vi "Autonomous Independent.vi"   [LabVIEW 2020]
doc: "This VI is called when autonomous begins, and will automatically be terminated when autonomous ends. You can carry out timed or sensor driven robot movement independently without needing to return to the caller."
uses:
  <vilib>/Rock Robotics/WPI/Utilities/WPI_GetSetVariantRefNum.vi
  <vilib>/Rock Robotics/Network Tables/NT Read String.vi
  <vilib>/Rock Robotics/Network Tables/NT Write Numeric Array.vi
  <vilib>/Rock Robotics/WPI/RobotDrive/WPI_RobotDriveArcadeDrive_Standard(NoSaturation).vi
panel:
  # "Be sure to right-click and choose Data Operations>>Make Current Value default if you want to save the array values with the VI"
types:
  T1 = typedef "WPI_JoystickDevRef.ctl" = cluster{"Device":T2}
  T2 = typedef "WPI_JoystickDeviceEnum.ctl" = enum16{"USB 0", "USB 1", "USB 2", "USB 3", "USB 4", "USB 5"}
  T3 = typedef "WPI_RobotDriveDevRef.ctl" = cluster{"DevStatus":errorcluster, "Motors[]":T4[], "Square Inputs":bool, "Max Output":dbl}
  T4 = typedef "WPI_MotorControlDeviceRef.ctl" = cluster{"DeviceStatus":errorcluster, "Type":T5, "PWM":cluster{"PWM Channel":T6, "DeadBand":T7}, "CAN":cluster{"Device Number":u8, "SetOutput VI Ref":variant, "GetOutput VI Ref":variant, "Enable VI Ref":variant, "Disable VI Ref":variant, "Data":variant}, "Invert":bool, "DIO PWM":cluster{"PWM \"Enable\" Channel":T6, "DIOChannel":T8, "PWM Rate":dbl}}
  T5 = typedef "WPI_MotorControlType.ctl" = enum16{"PWM", "CAN", "DIO PWM"}
  T6 = typedef "FPGA_DIOPWMChannel.ctl" = enum8{"PWM 0", "PWM 1", "PWM 2", "PWM 3", "PWM 4", "PWM 5", "PWM 6", "PWM 7", "PWM 8", "PWM 9", "PWM MXP 0", "PWM MXP 1", "PWM MXP 2", "PWM MXP 3", "PWM MXP 4", "PWM MXP 5", "PWM MXP 6", "PWM MXP 7", "PWM MXP 8", "PWM MXP 9", "Invalid"}
  T7 = typedef "WPI_PWMDeadband.ctl" = cluster{"Name":string, "maxPositivePwm":i32, "minPositivePwm":i32, "centerPwm":i32, "maxNegativePwm":i32, "minNegativePwm":i32, "angularRange":u16}
  T8 = typedef "FPGA_DIOChannel.ctl" = enum8{"DIO 0", "DIO 1", "DIO 2", "DIO 3", "DIO 4", "DIO 5", "DIO 6", "DIO 7", "DIO 8", "DIO 9", "DIO MXP 0", "DIO MXP 1", "DIO MXP 2", "DIO MXP 3", "DIO MXP 4", "DIO MXP 5", "DIO MXP 6", "DIO MXP 7", "DIO MXP 8", "DIO MXP 9", "DIO MXP 10", "DIO MXP 11", "DIO MXP 12", "DIO MXP 13", "DIO MXP 14", "DIO MXP 15", "SPI Port CS1", "SPI Port CS2", "SPI Port CS3", "SPI Port MISO", "SPI Port MOSI", "Invalid"}
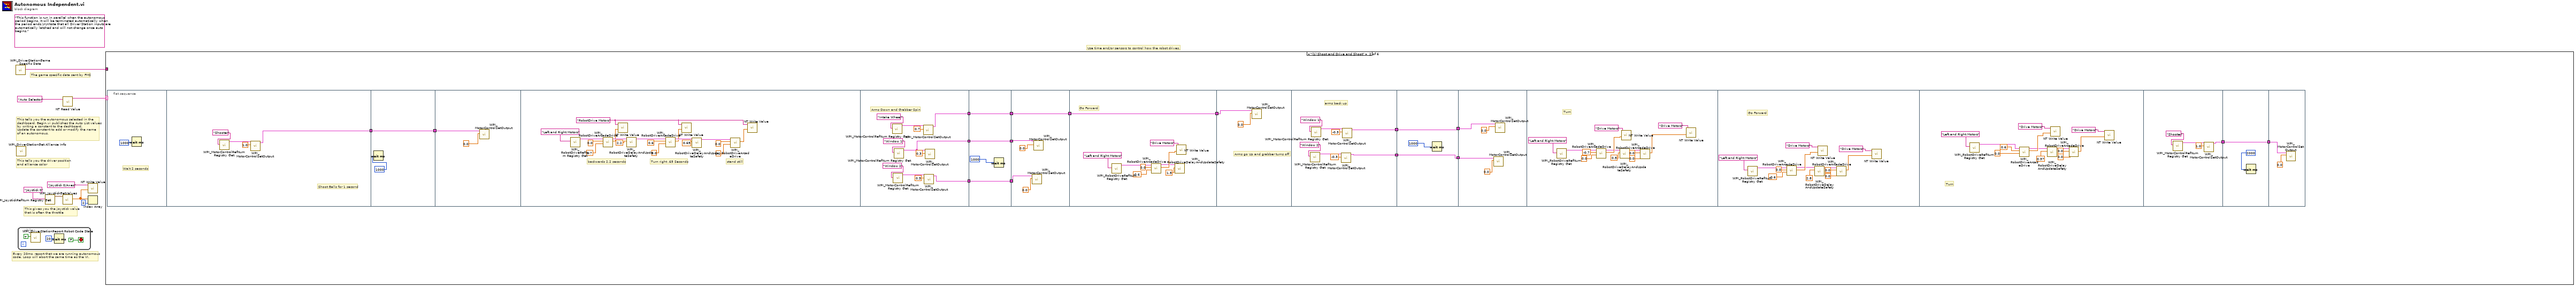
[diagram p0: block diagram]
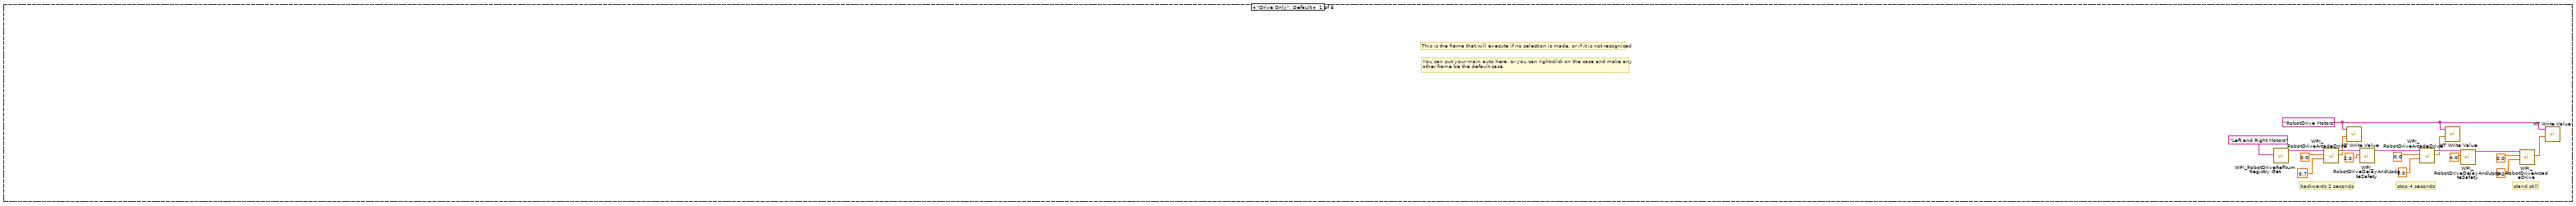
[diagram p2: hidden frame]
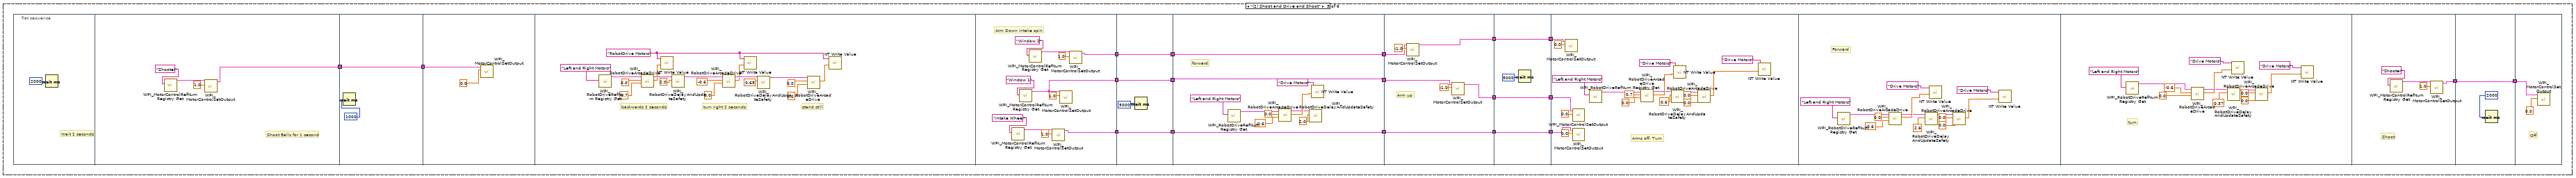
[diagram p3: hidden frame]
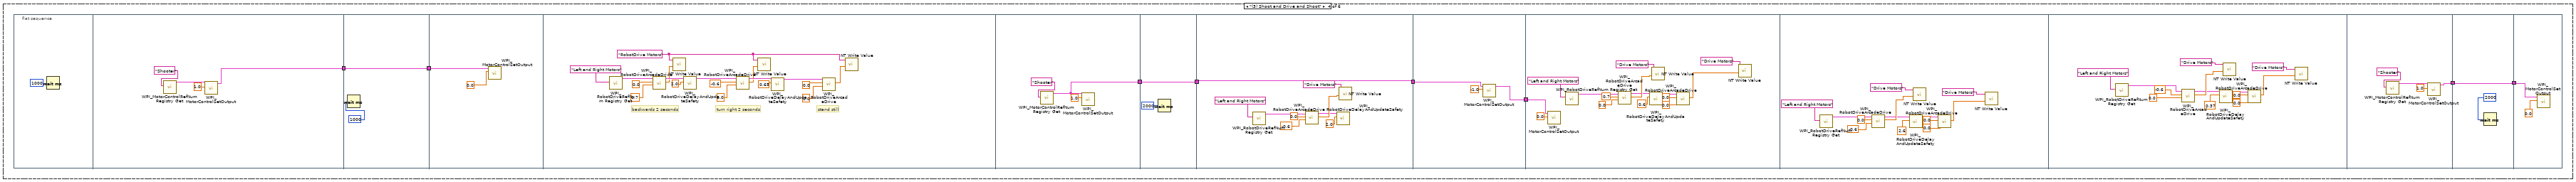
[diagram p4: hidden frame]
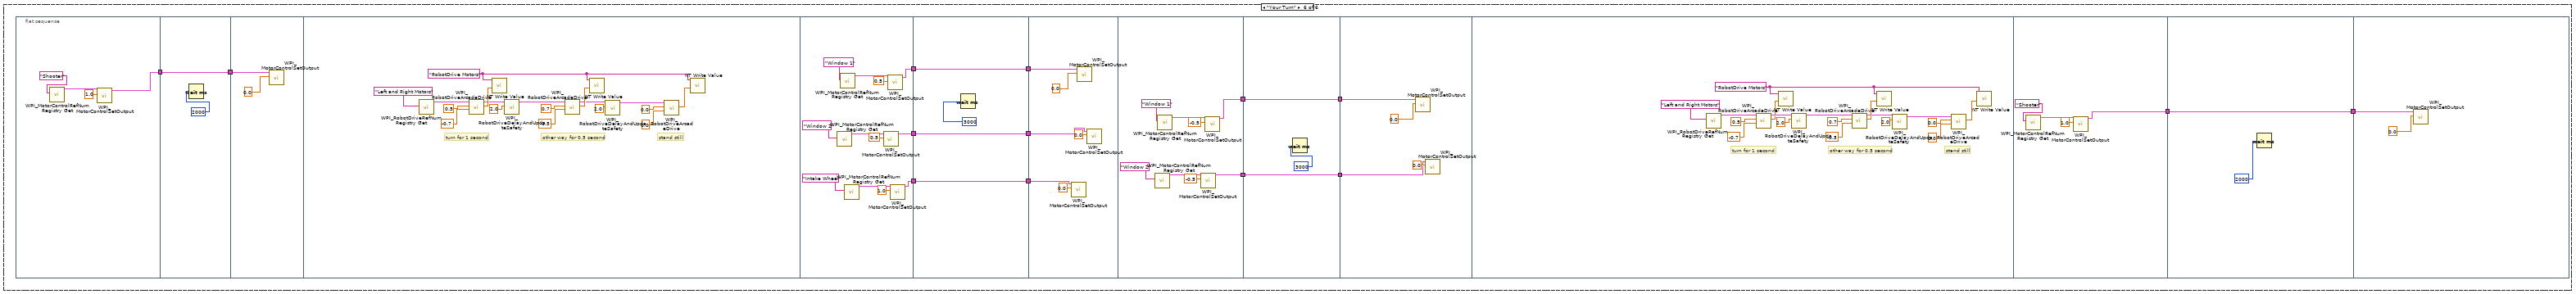
[diagram p6: hidden frame]
diagram:
  (unwired) "This function is run in parallel when the autonomous period begins. It will be terminated automatically when the period ends.\n\nNote that all Driver Station inputs are automatically latched and will not change once auto begins."
  # "The game specific data sent by FMS"
  # "This tells you the autonomous selected in the \ndashboard. Begin.vi publishes the Auto List values\nby writing a constant to the dashboard.\nUpdate the constant to add or modify the name\nof an autonomous."
  # "Every 20ms, report that we are running autonomous\ncode. Loop will abort the same time as the VI."
  # "This gives you the joystick value\nthat is often the throttle"
  # "Use time and/or sensors to control how the robot drives."
  # "This tells you the driver position\nand alliance color"
  n1 = call <vilib>:"WPI_DriverStationGame Specific Data.vi"() -> ("Game Specific Data"=w1:string)  [unwired: 11 in]
  n2 = call <vilib>:"WPI_DriverStationGet Alliance Info.vi"() -> ()  [unwired: 12 out]
  n3 = while {
    stop <- FALSE stop-if-true
    n4 = call <vilib>:"WPI_DriverStationReport Robot Code State.vi"("Autonomous"=TRUE) -> ()  [unwired: 10 in, 1 out]
    n5 = Wait (ms)(milliseconds to wait=u32 20) -> ()  [unwired: 1 out]
  }
  n6 = call <vilib>:"WPI_JoystickRefNum Registry Get.vi"("refnum name"="Joystick 0") -> ("JoystickDevRef"=w7:T1)  [unwired: 1 in, 9 out]
  n7 = call <vilib>:"WPI_JoystickGetValues.vi"("JoystickDevRef"=w7) -> ("Axes"=w3:dbl[])  [unwired: 6 in, 4 out]
  n8 = call-poly <vilib>:"NT Read Value.vi"("Name"="Auto Selector") -> ("String"=w4:string)  [unwired: 9 in, 1 out]
  n9 = call-poly <vilib>:"NT Write Value.vi"("Numeric Array"=w3, "Name"="Joystick 0/Axes") -> ()  [unwired: 9 in, 1 out]
  n10 = Index Array(array=w3, index=2) -> ()  [unwired: 1 out]
  n11 = case shown="\"(1) Shoot and Drive and Shoot\"" w4 {
    tunnel: w1 -> [_ _ _ _ _ _]
    frame "Drive Only", Default {
      w14 = "RobotDrive Motors" ("Name")
      # "stand still"
      # "stop 4 seconds"
      # "backwards 2 seconds"
      # "You can put your main auto here, or you can right-click on the case and make any\nother frame be the default case."
      # "This is the frame that will execute if no selection is made, or if it is not recognized"
      n12 = call <vilib>:"WPI_RobotDriveRefNum Registry Get.vi"("refnum name"="Left and Right Motors") -> ("RobotDriveDevRef"=w29:T3)  [unwired: 1 in, 9 out]
      n13 = call-poly <vilib>:"WPI_RobotDriveArcadeDrive.vi"("Y axis value"=0.7 ("X axis value"), "X axis value"=0.0, "RobotDriveDevRef"=w29) -> ("Motor Values"=w13:dbl[], "RobotDriveDevRef"=w23:T3)  [unwired: 1 in, 6 out]
      n14 = call-poly <vilib>:"NT Write Value.vi"("Numeric Array"=w13, "Name"=w14) -> ()  [unwired: 9 in, 1 out]
      n15 = call <vilib>:"WPI_RobotDriveDelayAndUpdateSafety.vi"("Delay (s)"=2.0, "RobotDriveDevRef"=w23) -> ("RobotDriveDevRef 2"=w12:T3)  [unwired: 8 in, 1 out]
      n16 = call-poly <vilib>:"WPI_RobotDriveArcadeDrive.vi"("Y axis value"=0.0 ("X axis value"), "X axis value"=0.0, "RobotDriveDevRef"=w12) -> ("Motor Values"=w15:dbl[], "RobotDriveDevRef"=w24:T3)  [unwired: 1 in, 6 out]
      n17 = call-poly <vilib>:"NT Write Value.vi"("Numeric Array"=w15, "Name"=w14) -> ()  [unwired: 9 in, 1 out]
      n18 = call <vilib>:"WPI_RobotDriveDelayAndUpdateSafety.vi"("Delay (s)"=4.0, "RobotDriveDevRef"=w24) -> ("RobotDriveDevRef 2"=w25:T3)  [unwired: 8 in, 1 out]
      n19 = call-poly <vilib>:"WPI_RobotDriveArcadeDrive.vi"("Y axis value"=0.0 ("X axis value"), "X axis value"=0.0, "RobotDriveDevRef"=w25) -> ("Motor Values"=w16:dbl[])  [unwired: 1 in, 7 out]
      n20 = call-poly <vilib>:"NT Write Value.vi"("Numeric Array"=w16, "Name"=w14) -> ()  [unwired: 9 in, 1 out]
    }
    frame "(1) Shoot and Drive and Shoot" {
      n21 = flat-sequence {
        tunnel: [w47] -> w45
        tunnel: w45 -> [w51]
        tunnel: [w51] -> w44
        tunnel: w44 -> [w53]
        tunnel: [w81] -> w43
        tunnel: [w77] -> w40
        tunnel: [w73] -> w38
        tunnel: w43 -> [w85]
        tunnel: w40 -> [w84]
        tunnel: [w86] -> w37
        tunnel: w38 -> [w86]
        tunnel: [w85] -> w35
        tunnel: [w84] -> w34
        tunnel: w37 -> [w92]
        tunnel: [w92] -> w36
        tunnel: w35 -> [w91]
        tunnel: w34 -> [w89]
        tunnel: [w93] -> w39
        tunnel: w36 -> [w93]
        tunnel: w39 -> [w103]
        tunnel: [w105] -> w32
        tunnel: [w104] -> w31
        tunnel: [w113] -> w33
        tunnel: w32 -> [w113]
        tunnel: w31 -> [w112]
        tunnel: [w112] -> w30
        tunnel: w33 -> [w116]
        tunnel: w30 -> [w115]
        tunnel: [w158] -> w41
        tunnel: [w162] -> w42
        tunnel: w41 -> [w162]
        tunnel: w42 -> [w164]
        frame #0 {
          # "Wait 2 seconds"
          n22 = Wait (ms)(milliseconds to wait=u32 1000) -> ()  [unwired: 1 out]
        }
        frame #1 {
          # "Shoot Balls for 1 second"
          n23 = call <vilib>:"WPI_MotorControlRefNum Registry Get.vi"("refnum name"="Shooter") -> ("MotorControlDevRef"=w50:T4)  [unwired: 9 in, 1 out]
          n24 = call <vilib>:"WPI_MotorControlSetOutput.vi"("Output"=1.0, "MotorControlDevRef"=w50) -> ("MotorControlDevRef"=w47:T4)  [unwired: 7 in, 2 out]
        }
        frame #2 {
          n25 = Wait (ms)(milliseconds to wait=u32 1000) -> ()  [unwired: 1 out]
        }
        frame #3 {
          n26 = call <vilib>:"WPI_MotorControlSetOutput.vi"("Output"=0.0, "MotorControlDevRef"=w53) -> ()  [unwired: 7 in, 3 out]
        }
        frame #4 {
          w57 = "RobotDrive Motors" ("Name")
          # "stand still"
          # "Turn right .65 Seconds"
          # "backwards 2.2 seconds"
          n27 = call <vilib>:"WPI_RobotDriveRefNum Registry Get.vi"("refnum name"="Left and Right Motors") -> ("RobotDriveDevRef"=w72:T3)  [unwired: 1 in, 9 out]
          n28 = call-poly <vilib>:"WPI_RobotDriveArcadeDrive.vi"("Y axis value"=0.7 ("X axis value"), "X axis value"=0.0, "RobotDriveDevRef"=w72) -> ("Motor Values"=w56:dbl[], "RobotDriveDevRef"=w66:T3)  [unwired: 1 in, 6 out]
          n29 = call-poly <vilib>:"NT Write Value.vi"("Numeric Array"=w56, "Name"=w57) -> ()  [unwired: 9 in, 1 out]
          n30 = call <vilib>:"WPI_RobotDriveDelayAndUpdateSafety.vi"("Delay (s)"=2.2, "RobotDriveDevRef"=w66) -> ("RobotDriveDevRef 2"=w55:T3)  [unwired: 8 in, 1 out]
          n31 = call-poly <vilib>:"WPI_RobotDriveArcadeDrive.vi"("Y axis value"=0.0 ("X axis value"), "X axis value"=0.6, "RobotDriveDevRef"=w55) -> ("Motor Values"=w58:dbl[], "RobotDriveDevRef"=w67:T3)  [unwired: 1 in, 6 out]
          n32 = call-poly <vilib>:"NT Write Value.vi"("Numeric Array"=w58, "Name"=w57) -> ()  [unwired: 9 in, 1 out]
          n33 = call <vilib>:"WPI_RobotDriveDelayAndUpdateSafety.vi"("Delay (s)"=0.65, "RobotDriveDevRef"=w67) -> ("RobotDriveDevRef 2"=w68:T3)  [unwired: 8 in, 1 out]
          n34 = call-poly <vilib>:"WPI_RobotDriveArcadeDrive.vi"("Y axis value"=0.0 ("X axis value"), "X axis value"=0.0, "RobotDriveDevRef"=w68) -> ("Motor Values"=w59:dbl[])  [unwired: 1 in, 7 out]
          n35 = call-poly <vilib>:"NT Write Value.vi"("Numeric Array"=w59, "Name"=w57) -> ()  [unwired: 9 in, 1 out]
        }
        frame #5 {
          # "Arms Down and Grabber Spin"
          n36 = call <vilib>:"WPI_MotorControlRefNum Registry Get.vi"("refnum name"="Intake Wheel") -> ("MotorControlDevRef"=w74:T4)  [unwired: 9 in, 1 out]
          n37 = call <vilib>:"WPI_MotorControlRefNum Registry Get.vi"("refnum name"="Window 2") -> ("MotorControlDevRef"=w79:T4)  [unwired: 9 in, 1 out]
          n38 = call <vilib>:"WPI_MotorControlRefNum Registry Get.vi"("refnum name"="Window 1") -> ("MotorControlDevRef"=w81:T4)  [unwired: 9 in, 1 out]
          n39 = call <vilib>:"WPI_MotorControlSetOutput.vi"("Output"=0.7, "MotorControlDevRef"=w74) -> ("MotorControlDevRef"=w73:T4)  [unwired: 7 in, 2 out]
          n40 = call <vilib>:"WPI_MotorControlSetOutput.vi"("Output"=0.3, "MotorControlDevRef"=w79) -> ("MotorControlDevRef"=w77:T4)  [unwired: 7 in, 2 out]
          n41 = call <vilib>:"WPI_MotorControlSetOutput.vi"("Output"=0.3, "MotorControlDevRef"=w81) -> ()  [unwired: 7 in, 3 out]
        }
        frame #6 {
          n42 = Wait (ms)(milliseconds to wait=u32 1000) -> ()  [unwired: 1 out]
        }
        frame #7 {
          n43 = call <vilib>:"WPI_MotorControlSetOutput.vi"("Output"=0.0, "MotorControlDevRef"=w89) -> ()  [unwired: 7 in, 3 out]
          n44 = call <vilib>:"WPI_MotorControlSetOutput.vi"("Output"=0.0, "MotorControlDevRef"=w91) -> ()  [unwired: 7 in, 3 out]
        }
        frame #8 {
          # "Go Forward"
          n45 = call <vilib>:"WPI_RobotDriveRefNum Registry Get.vi"("refnum name"="Left and Right Motors") -> ("RobotDriveDevRef"=w101:T3)  [unwired: 9 in, 1 out]
          n46 = call-poly <vilib>:"WPI_RobotDriveArcadeDrive.vi"("Y axis value"=-0.6, "X axis value"=0.0, "RobotDriveDevRef"=w101) -> ("Motor Values"=w100:dbl[], "RobotDriveDevRef"=w97:T3)  [unwired: 6 in, 1 out]
          n47 = call <vilib>:"WPI_RobotDriveDelayAndUpdateSafety.vi"("Delay (s)"=1.5, "RobotDriveDevRef"=w97) -> ()  [unwired: 8 in, 2 out]
          n48 = call-poly <vilib>:"NT Write Value.vi"("Numeric Array"=w100, "Name"="Drive Motors") -> ()  [unwired: 9 in, 1 out]
        }
        frame #9 {
          # "Arms go Up and grabber turns off"
          n49 = call <vilib>:"WPI_MotorControlSetOutput.vi"("Output"=0.0, "MotorControlDevRef"=w103) -> ()  [unwired: 7 in, 3 out]
        }
        frame #10 {
          # "arms back up"
          n50 = call <vilib>:"WPI_MotorControlRefNum Registry Get.vi"("refnum name"="Window 2") -> ("MotorControlDevRef"=w107:T4)  [unwired: 9 in, 1 out]
          n51 = call <vilib>:"WPI_MotorControlRefNum Registry Get.vi"("refnum name"="Window 1") -> ("MotorControlDevRef"=w109:T4)  [unwired: 9 in, 1 out]
          n52 = call <vilib>:"WPI_MotorControlSetOutput.vi"("Output"=-0.3, "MotorControlDevRef"=w107) -> ("MotorControlDevRef"=w104:T4)  [unwired: 7 in, 2 out]
          n53 = call <vilib>:"WPI_MotorControlSetOutput.vi"("Output"=-0.3, "MotorControlDevRef"=w109) -> ("MotorControlDevRef"=w105:T4)  [unwired: 7 in, 2 out]
        }
        frame #11 {
          n54 = Wait (ms)(milliseconds to wait=u32 1000) -> ()  [unwired: 1 out]
        }
        frame #12 {
          n55 = call <vilib>:"WPI_MotorControlSetOutput.vi"("Output"=0.0, "MotorControlDevRef"=w115) -> ()  [unwired: 7 in, 3 out]
          n56 = call <vilib>:"WPI_MotorControlSetOutput.vi"("Output"=0.0, "MotorControlDevRef"=w116) -> ()  [unwired: 7 in, 3 out]
        }
        frame #13 {
          # "Turn"
          n57 = call <vilib>:"WPI_RobotDriveRefNum Registry Get.vi"("refnum name"="Left and Right Motors") -> ("RobotDriveDevRef"=w131:T3)  [unwired: 9 in, 1 out]
          n58 = call-poly <vilib>:"WPI_RobotDriveArcadeDrive.vi"("Y axis value"=0.0, "X axis value"=-0.7, "RobotDriveDevRef"=w131) -> ("Motor Values"=w130:dbl[], "RobotDriveDevRef"=w128:T3)  [unwired: 6 in, 1 out]
          n59 = call <vilib>:"WPI_RobotDriveDelayAndUpdateSafety.vi"("Delay (s)"=0.5, "RobotDriveDevRef"=w128) -> ("RobotDriveDevRef 2"=w124:T3)  [unwired: 8 in, 1 out]
          n60 = call-poly <vilib>:"NT Write Value.vi"("Numeric Array"=w130, "Name"="Drive Motors") -> ()  [unwired: 9 in, 1 out]
          n61 = call-poly <vilib>:"WPI_RobotDriveArcadeDrive.vi"("Y axis value"=0.0, "X axis value"=0.0, "RobotDriveDevRef"=w124) -> ("Motor Values"=w121:dbl[])  [unwired: 6 in, 2 out]
          n62 = call-poly <vilib>:"NT Write Value.vi"("Numeric Array"=w121, "Name"="Drive Motors") -> ()  [unwired: 9 in, 1 out]
        }
        frame #14 {
          # "Go Forward"
          n63 = call <vilib>:"WPI_RobotDriveRefNum Registry Get.vi"("refnum name"="Left and Right Motors") -> ("RobotDriveDevRef"=w144:T3)  [unwired: 9 in, 1 out]
          n64 = call-poly <vilib>:"WPI_RobotDriveArcadeDrive.vi"("Y axis value"=-0.6, "X axis value"=0.0, "RobotDriveDevRef"=w144) -> ("Motor Values"=w143:dbl[], "RobotDriveDevRef"=w141:T3)  [unwired: 6 in, 1 out]
          n65 = call <vilib>:"WPI_RobotDriveDelayAndUpdateSafety.vi"("Delay (s)"=2.8, "RobotDriveDevRef"=w141) -> ("RobotDriveDevRef 2"=w136:T3)  [unwired: 8 in, 1 out]
          n66 = call-poly <vilib>:"NT Write Value.vi"("Numeric Array"=w143, "Name"="Drive Motors") -> ()  [unwired: 9 in, 1 out]
          n67 = call-poly <vilib>:"WPI_RobotDriveArcadeDrive.vi"("Y axis value"=0.0, "X axis value"=0.0, "RobotDriveDevRef"=w136) -> ("Motor Values"=w132:dbl[])  [unwired: 6 in, 2 out]
          n68 = call-poly <vilib>:"NT Write Value.vi"("Numeric Array"=w132, "Name"="Drive Motors") -> ()  [unwired: 9 in, 1 out]
        }
        frame #15 {
          # "Turn"
          n69 = call <vilib>:"WPI_RobotDriveRefNum Registry Get.vi"("refnum name"="Left and Right Motors") -> ("RobotDriveDevRef"=w157:T3)  [unwired: 9 in, 1 out]
          n70 = call-poly <vilib>:"WPI_RobotDriveArcadeDrive.vi"("Y axis value"=0.0, "X axis value"=0.6, "RobotDriveDevRef"=w157) -> ("Motor Values"=w156:dbl[], "RobotDriveDevRef"=w154:T3)  [unwired: 6 in, 1 out]
          n71 = call <vilib>:"WPI_RobotDriveDelayAndUpdateSafety.vi"("Delay (s)"=0.37, "RobotDriveDevRef"=w154) -> ("RobotDriveDevRef 2"=w149:T3)  [unwired: 8 in, 1 out]
          n72 = call-poly <vilib>:"NT Write Value.vi"("Numeric Array"=w156, "Name"="Drive Motors") -> ()  [unwired: 9 in, 1 out]
          n73 = call-poly <vilib>:"WPI_RobotDriveArcadeDrive.vi"("Y axis value"=0.0, "X axis value"=0.0, "RobotDriveDevRef"=w149) -> ("Motor Values"=w145:dbl[])  [unwired: 6 in, 2 out]
          n74 = call-poly <vilib>:"NT Write Value.vi"("Numeric Array"=w145, "Name"="Drive Motors") -> ()  [unwired: 9 in, 1 out]
        }
        frame #16 {
          n75 = call <vilib>:"WPI_MotorControlRefNum Registry Get.vi"("refnum name"="Shooter") -> ("MotorControlDevRef"=w161:T4)  [unwired: 9 in, 1 out]
          n76 = call <vilib>:"WPI_MotorControlSetOutput.vi"("Output"=1.0, "MotorControlDevRef"=w161) -> ("MotorControlDevRef"=w158:T4)  [unwired: 7 in, 2 out]
        }
        frame #17 {
          n77 = Wait (ms)(milliseconds to wait=u32 2000) -> ()  [unwired: 1 out]
        }
        frame #18 {
          n78 = call <vilib>:"WPI_MotorControlSetOutput.vi"("Output"=0.0, "MotorControlDevRef"=w164) -> ()  [unwired: 7 in, 3 out]
        }
      }
    }
    frame "(2) Shoot and Drive and Shoot" {
      n79 = flat-sequence {
        tunnel: [w186] -> w184
        tunnel: w184 -> [w190]
        tunnel: [w190] -> w183
        tunnel: w183 -> [w192]
        tunnel: [w220] -> w181
        tunnel: [w216] -> w175
        tunnel: [w212] -> w172
        tunnel: w181 -> [w226]
        tunnel: [w226] -> w180
        tunnel: [w224] -> w176
        tunnel: w175 -> [w224]
        tunnel: [w223] -> w173
        tunnel: w172 -> [w223]
        tunnel: [w237] -> w182
        tunnel: w180 -> [w237]
        tunnel: [w228] -> w177
        tunnel: w176 -> [w228]
        tunnel: [w227] -> w174
        tunnel: w173 -> [w227]
        tunnel: w182 -> [w243]
        tunnel: [w242] -> w171
        tunnel: w177 -> [w240]
        tunnel: [w239] -> w169
        tunnel: [w238] -> w167
        tunnel: w174 -> [w238]
        tunnel: w171 -> [w248]
        tunnel: [w248] -> w170
        tunnel: w169 -> [w247]
        tunnel: [w247] -> w168
        tunnel: w167 -> [w246]
        tunnel: [w246] -> w166
        tunnel: w170 -> [w253]
        tunnel: w168 -> [w251]
        tunnel: w166 -> [w249]
        tunnel: [w294] -> w178
        tunnel: [w298] -> w179
        tunnel: w178 -> [w298]
        tunnel: w179 -> [w300]
        frame #0 {
          # "Wait 2 seconds"
          n80 = Wait (ms)(milliseconds to wait=u32 2000) -> ()  [unwired: 1 out]
        }
        frame #1 {
          # "Shoot Balls for 1 second"
          n81 = call <vilib>:"WPI_MotorControlRefNum Registry Get.vi"("refnum name"="Shooter") -> ("MotorControlDevRef"=w189:T4)  [unwired: 9 in, 1 out]
          n82 = call <vilib>:"WPI_MotorControlSetOutput.vi"("Output"=1.0, "MotorControlDevRef"=w189) -> ("MotorControlDevRef"=w186:T4)  [unwired: 7 in, 2 out]
        }
        frame #2 {
          n83 = Wait (ms)(milliseconds to wait=u32 1000) -> ()  [unwired: 1 out]
        }
        frame #3 {
          n84 = call <vilib>:"WPI_MotorControlSetOutput.vi"("Output"=0.0, "MotorControlDevRef"=w192) -> ()  [unwired: 7 in, 3 out]
        }
        frame #4 {
          w196 = "RobotDrive Motors" ("Name")
          # "stand still"
          # "turn right 2 seconds"
          # "backwards 2 seconds"
          n85 = call <vilib>:"WPI_RobotDriveRefNum Registry Get.vi"("refnum name"="Left and Right Motors") -> ("RobotDriveDevRef"=w211:T3)  [unwired: 1 in, 9 out]
          n86 = call-poly <vilib>:"WPI_RobotDriveArcadeDrive.vi"("Y axis value"=0.7 ("X axis value"), "X axis value"=0.0, "RobotDriveDevRef"=w211) -> ("Motor Values"=w195:dbl[], "RobotDriveDevRef"=w205:T3)  [unwired: 1 in, 6 out]
          n87 = call-poly <vilib>:"NT Write Value.vi"("Numeric Array"=w195, "Name"=w196) -> ()  [unwired: 9 in, 1 out]
          n88 = call <vilib>:"WPI_RobotDriveDelayAndUpdateSafety.vi"("Delay (s)"=2.0, "RobotDriveDevRef"=w205) -> ("RobotDriveDevRef 2"=w194:T3)  [unwired: 8 in, 1 out]
          n89 = call-poly <vilib>:"WPI_RobotDriveArcadeDrive.vi"("Y axis value"=0.0 ("X axis value"), "X axis value"=-0.6, "RobotDriveDevRef"=w194) -> ("Motor Values"=w197:dbl[], "RobotDriveDevRef"=w206:T3)  [unwired: 1 in, 6 out]
          n90 = call-poly <vilib>:"NT Write Value.vi"("Numeric Array"=w197, "Name"=w196) -> ()  [unwired: 9 in, 1 out]
          n91 = call <vilib>:"WPI_RobotDriveDelayAndUpdateSafety.vi"("Delay (s)"=0.65, "RobotDriveDevRef"=w206) -> ("RobotDriveDevRef 2"=w207:T3)  [unwired: 8 in, 1 out]
          n92 = call-poly <vilib>:"WPI_RobotDriveArcadeDrive.vi"("Y axis value"=0.0 ("X axis value"), "X axis value"=0.0, "RobotDriveDevRef"=w207) -> ("Motor Values"=w198:dbl[])  [unwired: 1 in, 7 out]
          n93 = call-poly <vilib>:"NT Write Value.vi"("Numeric Array"=w198, "Name"=w196) -> ()  [unwired: 9 in, 1 out]
        }
        frame #5 {
          # "Arm Down Intake spin"
          n94 = call <vilib>:"WPI_MotorControlRefNum Registry Get.vi"("refnum name"="Intake Wheel") -> ("MotorControlDevRef"=w214:T4)  [unwired: 9 in, 1 out]
          n95 = call <vilib>:"WPI_MotorControlRefNum Registry Get.vi"("refnum name"="Window 1") -> ("MotorControlDevRef"=w220:T4)  [unwired: 9 in, 1 out]
          n96 = call <vilib>:"WPI_MotorControlRefNum Registry Get.vi"("refnum name"="Window 2") -> ("MotorControlDevRef"=w218:T4)  [unwired: 9 in, 1 out]
          n97 = call <vilib>:"WPI_MotorControlSetOutput.vi"("Output"=1.0, "MotorControlDevRef"=w214) -> ("MotorControlDevRef"=w212:T4)  [unwired: 7 in, 2 out]
          n98 = call <vilib>:"WPI_MotorControlSetOutput.vi"("Output"=1.0, "MotorControlDevRef"=w220) -> ()  [unwired: 7 in, 3 out]
          n99 = call <vilib>:"WPI_MotorControlSetOutput.vi"("Output"=1.0, "MotorControlDevRef"=w218) -> ("MotorControlDevRef"=w216:T4)  [unwired: 7 in, 2 out]
        }
        frame #6 {
          n100 = Wait (ms)(milliseconds to wait=u32 5000) -> ()  [unwired: 1 out]
        }
        frame #7 {
          # "forward"
          n101 = call <vilib>:"WPI_RobotDriveRefNum Registry Get.vi"("refnum name"="Left and Right Motors") -> ("RobotDriveDevRef"=w236:T3)  [unwired: 9 in, 1 out]
          n102 = call-poly <vilib>:"WPI_RobotDriveArcadeDrive.vi"("Y axis value"=-0.6, "X axis value"=0.0, "RobotDriveDevRef"=w236) -> ("Motor Values"=w235:dbl[], "RobotDriveDevRef"=w232:T3)  [unwired: 6 in, 1 out]
          n103 = call <vilib>:"WPI_RobotDriveDelayAndUpdateSafety.vi"("Delay (s)"=2.0, "RobotDriveDevRef"=w232) -> ()  [unwired: 8 in, 2 out]
          n104 = call-poly <vilib>:"NT Write Value.vi"("Numeric Array"=w235, "Name"="Drive Motors") -> ()  [unwired: 9 in, 1 out]
        }
        frame #8 {
          # "Arm up"
          n105 = call <vilib>:"WPI_MotorControlSetOutput.vi"("Output"=-1.0, "MotorControlDevRef"=w240) -> ("MotorControlDevRef"=w239:T4)  [unwired: 7 in, 2 out]
          n106 = call <vilib>:"WPI_MotorControlSetOutput.vi"("Output"=-1.0, "MotorControlDevRef"=w243) -> ("MotorControlDevRef"=w242:T4)  [unwired: 7 in, 2 out]
        }
        frame #9 {
          n107 = Wait (ms)(milliseconds to wait=u32 5000) -> ()  [unwired: 1 out]
        }
        frame #10 {
          # "Arms off, Turn"
          n108 = call <vilib>:"WPI_MotorControlSetOutput.vi"("Output"=0.0, "MotorControlDevRef"=w251) -> ()  [unwired: 7 in, 3 out]
          n109 = call <vilib>:"WPI_MotorControlSetOutput.vi"("Output"=0.0, "MotorControlDevRef"=w253) -> ()  [unwired: 7 in, 3 out]
          n110 = call <vilib>:"WPI_MotorControlSetOutput.vi"("Output"=0.0, "MotorControlDevRef"=w249) -> ()  [unwired: 7 in, 3 out]
          n111 = call <vilib>:"WPI_RobotDriveRefNum Registry Get.vi"("refnum name"="Left and Right Motors") -> ("RobotDriveDevRef"=w267:T3)  [unwired: 9 in, 1 out]
          n112 = call-poly <vilib>:"WPI_RobotDriveArcadeDrive.vi"("Y axis value"=0.0, "X axis value"=0.7, "RobotDriveDevRef"=w267) -> ("Motor Values"=w266:dbl[], "RobotDriveDevRef"=w264:T3)  [unwired: 6 in, 1 out]
          n113 = call <vilib>:"WPI_RobotDriveDelayAndUpdateSafety.vi"("Delay (s)"=0.6, "RobotDriveDevRef"=w264) -> ("RobotDriveDevRef 2"=w260:T3)  [unwired: 8 in, 1 out]
          n114 = call-poly <vilib>:"NT Write Value.vi"("Numeric Array"=w266, "Name"="Drive Motors") -> ()  [unwired: 9 in, 1 out]
          n115 = call-poly <vilib>:"WPI_RobotDriveArcadeDrive.vi"("Y axis value"=0.0, "X axis value"=0.0, "RobotDriveDevRef"=w260) -> ("Motor Values"=w257:dbl[])  [unwired: 6 in, 2 out]
          n116 = call-poly <vilib>:"NT Write Value.vi"("Numeric Array"=w257, "Name"="Drive Motors") -> ()  [unwired: 9 in, 1 out]
        }
        frame #11 {
          # "Forward"
          n117 = call <vilib>:"WPI_RobotDriveRefNum Registry Get.vi"("refnum name"="Left and Right Motors") -> ("RobotDriveDevRef"=w280:T3)  [unwired: 9 in, 1 out]
          n118 = call-poly <vilib>:"WPI_RobotDriveArcadeDrive.vi"("Y axis value"=-0.6, "X axis value"=0.0, "RobotDriveDevRef"=w280) -> ("Motor Values"=w279:dbl[], "RobotDriveDevRef"=w277:T3)  [unwired: 6 in, 1 out]
          n119 = call <vilib>:"WPI_RobotDriveDelayAndUpdateSafety.vi"("Delay (s)"=2.6, "RobotDriveDevRef"=w277) -> ("RobotDriveDevRef 2"=w272:T3)  [unwired: 8 in, 1 out]
          n120 = call-poly <vilib>:"NT Write Value.vi"("Numeric Array"=w279, "Name"="Drive Motors") -> ()  [unwired: 9 in, 1 out]
          n121 = call-poly <vilib>:"WPI_RobotDriveArcadeDrive.vi"("Y axis value"=0.0, "X axis value"=0.0, "RobotDriveDevRef"=w272) -> ("Motor Values"=w268:dbl[])  [unwired: 6 in, 2 out]
          n122 = call-poly <vilib>:"NT Write Value.vi"("Numeric Array"=w268, "Name"="Drive Motors") -> ()  [unwired: 9 in, 1 out]
        }
        frame #12 {
          # "turn"
          n123 = call <vilib>:"WPI_RobotDriveRefNum Registry Get.vi"("refnum name"="Left and Right Motors") -> ("RobotDriveDevRef"=w293:T3)  [unwired: 9 in, 1 out]
          n124 = call-poly <vilib>:"WPI_RobotDriveArcadeDrive.vi"("Y axis value"=0.0, "X axis value"=-0.6, "RobotDriveDevRef"=w293) -> ("Motor Values"=w292:dbl[], "RobotDriveDevRef"=w290:T3)  [unwired: 6 in, 1 out]
          n125 = call <vilib>:"WPI_RobotDriveDelayAndUpdateSafety.vi"("Delay (s)"=0.37, "RobotDriveDevRef"=w290) -> ("RobotDriveDevRef 2"=w285:T3)  [unwired: 8 in, 1 out]
          n126 = call-poly <vilib>:"NT Write Value.vi"("Numeric Array"=w292, "Name"="Drive Motors") -> ()  [unwired: 9 in, 1 out]
          n127 = call-poly <vilib>:"WPI_RobotDriveArcadeDrive.vi"("Y axis value"=0.0, "X axis value"=0.0, "RobotDriveDevRef"=w285) -> ("Motor Values"=w281:dbl[])  [unwired: 6 in, 2 out]
          n128 = call-poly <vilib>:"NT Write Value.vi"("Numeric Array"=w281, "Name"="Drive Motors") -> ()  [unwired: 9 in, 1 out]
        }
        frame #13 {
          # "Shoot"
          n129 = call <vilib>:"WPI_MotorControlRefNum Registry Get.vi"("refnum name"="Shooter") -> ("MotorControlDevRef"=w297:T4)  [unwired: 9 in, 1 out]
          n130 = call <vilib>:"WPI_MotorControlSetOutput.vi"("Output"=1.0, "MotorControlDevRef"=w297) -> ("MotorControlDevRef"=w294:T4)  [unwired: 7 in, 2 out]
        }
        frame #14 {
          n131 = Wait (ms)(milliseconds to wait=u32 2000) -> ()  [unwired: 1 out]
        }
        frame #15 {
          # "Off"
          n132 = call <vilib>:"WPI_MotorControlSetOutput.vi"("Output"=0.0, "MotorControlDevRef"=w300) -> ()  [unwired: 7 in, 3 out]
        }
      }
    }
    frame "(3) Shoot and Drive and Shoot" {
      n133 = flat-sequence {
        tunnel: [w311] -> w309
        tunnel: w309 -> [w315]
        tunnel: [w315] -> w308
        tunnel: w308 -> [w317]
        tunnel: [w337] -> w305
        tunnel: w305 -> [w341]
        tunnel: [w341] -> w304
        tunnel: [w350] -> w307
        tunnel: w304 -> [w350]
        tunnel: w307 -> [w352]
        tunnel: [w351] -> w306
        tunnel: w306 -> [w354]
        tunnel: [w395] -> w302
        tunnel: [w399] -> w303
        tunnel: w302 -> [w399]
        tunnel: w303 -> [w401]
        frame #0 {
          n134 = Wait (ms)(milliseconds to wait=u32 1000) -> ()  [unwired: 1 out]
        }
        frame #1 {
          n135 = call <vilib>:"WPI_MotorControlRefNum Registry Get.vi"("refnum name"="Shooter") -> ("MotorControlDevRef"=w314:T4)  [unwired: 9 in, 1 out]
          n136 = call <vilib>:"WPI_MotorControlSetOutput.vi"("Output"=1.0, "MotorControlDevRef"=w314) -> ("MotorControlDevRef"=w311:T4)  [unwired: 7 in, 2 out]
        }
        frame #2 {
          n137 = Wait (ms)(milliseconds to wait=u32 1000) -> ()  [unwired: 1 out]
        }
        frame #3 {
          n138 = call <vilib>:"WPI_MotorControlSetOutput.vi"("Output"=0.0, "MotorControlDevRef"=w317) -> ()  [unwired: 7 in, 3 out]
        }
        frame #4 {
          w321 = "RobotDrive Motors" ("Name")
          # "stand still"
          # "turn right 2 seconds"
          # "backwards 2 seconds"
          n139 = call <vilib>:"WPI_RobotDriveRefNum Registry Get.vi"("refnum name"="Left and Right Motors") -> ("RobotDriveDevRef"=w336:T3)  [unwired: 1 in, 9 out]
          n140 = call-poly <vilib>:"WPI_RobotDriveArcadeDrive.vi"("Y axis value"=0.7 ("X axis value"), "X axis value"=0.0, "RobotDriveDevRef"=w336) -> ("Motor Values"=w320:dbl[], "RobotDriveDevRef"=w330:T3)  [unwired: 1 in, 6 out]
          n141 = call-poly <vilib>:"NT Write Value.vi"("Numeric Array"=w320, "Name"=w321) -> ()  [unwired: 9 in, 1 out]
          n142 = call <vilib>:"WPI_RobotDriveDelayAndUpdateSafety.vi"("Delay (s)"=2.0, "RobotDriveDevRef"=w330) -> ("RobotDriveDevRef 2"=w319:T3)  [unwired: 8 in, 1 out]
          n143 = call-poly <vilib>:"WPI_RobotDriveArcadeDrive.vi"("Y axis value"=0.0 ("X axis value"), "X axis value"=-0.6, "RobotDriveDevRef"=w319) -> ("Motor Values"=w322:dbl[], "RobotDriveDevRef"=w331:T3)  [unwired: 1 in, 6 out]
          n144 = call-poly <vilib>:"NT Write Value.vi"("Numeric Array"=w322, "Name"=w321) -> ()  [unwired: 9 in, 1 out]
          n145 = call <vilib>:"WPI_RobotDriveDelayAndUpdateSafety.vi"("Delay (s)"=0.65, "RobotDriveDevRef"=w331) -> ("RobotDriveDevRef 2"=w332:T3)  [unwired: 8 in, 1 out]
          n146 = call-poly <vilib>:"WPI_RobotDriveArcadeDrive.vi"("Y axis value"=0.0 ("X axis value"), "X axis value"=0.0, "RobotDriveDevRef"=w332) -> ("Motor Values"=w323:dbl[])  [unwired: 1 in, 7 out]
          n147 = call-poly <vilib>:"NT Write Value.vi"("Numeric Array"=w323, "Name"=w321) -> ()  [unwired: 9 in, 1 out]
        }
        frame #5 {
          n148 = call <vilib>:"WPI_MotorControlRefNum Registry Get.vi"("refnum name"="Shooter") -> ("MotorControlDevRef"=w337:T4)  [unwired: 9 in, 1 out]
          n149 = call <vilib>:"WPI_MotorControlSetOutput.vi"("Output"=1.0, "MotorControlDevRef"=w337) -> ()  [unwired: 7 in, 3 out]
        }
        frame #6 {
          n150 = Wait (ms)(milliseconds to wait=u32 2000) -> ()  [unwired: 1 out]
        }
        frame #7 {
          n151 = call <vilib>:"WPI_RobotDriveRefNum Registry Get.vi"("refnum name"="Left and Right Motors") -> ("RobotDriveDevRef"=w349:T3)  [unwired: 9 in, 1 out]
          n152 = call-poly <vilib>:"WPI_RobotDriveArcadeDrive.vi"("Y axis value"=-0.6, "X axis value"=0.0, "RobotDriveDevRef"=w349) -> ("Motor Values"=w348:dbl[], "RobotDriveDevRef"=w345:T3)  [unwired: 6 in, 1 out]
          n153 = call <vilib>:"WPI_RobotDriveDelayAndUpdateSafety.vi"("Delay (s)"=2.0, "RobotDriveDevRef"=w345) -> ()  [unwired: 8 in, 2 out]
          n154 = call-poly <vilib>:"NT Write Value.vi"("Numeric Array"=w348, "Name"="Drive Motors") -> ()  [unwired: 9 in, 1 out]
        }
        frame #8 {
          n155 = call <vilib>:"WPI_MotorControlSetOutput.vi"("Output"=-1.0, "MotorControlDevRef"=w352) -> ("MotorControlDevRef"=w351:T4)  [unwired: 7 in, 2 out]
        }
        frame #9 {
          n156 = call <vilib>:"WPI_MotorControlSetOutput.vi"("Output"=0.0, "MotorControlDevRef"=w354) -> ()  [unwired: 7 in, 3 out]
          n157 = call <vilib>:"WPI_RobotDriveRefNum Registry Get.vi"("refnum name"="Left and Right Motors") -> ("RobotDriveDevRef"=w368:T3)  [unwired: 9 in, 1 out]
          n158 = call-poly <vilib>:"WPI_RobotDriveArcadeDrive.vi"("Y axis value"=0.0, "X axis value"=0.7, "RobotDriveDevRef"=w368) -> ("Motor Values"=w367:dbl[], "RobotDriveDevRef"=w365:T3)  [unwired: 6 in, 1 out]
          n159 = call <vilib>:"WPI_RobotDriveDelayAndUpdateSafety.vi"("Delay (s)"=0.6, "RobotDriveDevRef"=w365) -> ("RobotDriveDevRef 2"=w361:T3)  [unwired: 8 in, 1 out]
          n160 = call-poly <vilib>:"NT Write Value.vi"("Numeric Array"=w367, "Name"="Drive Motors") -> ()  [unwired: 9 in, 1 out]
          n161 = call-poly <vilib>:"WPI_RobotDriveArcadeDrive.vi"("Y axis value"=0.0, "X axis value"=0.0, "RobotDriveDevRef"=w361) -> ("Motor Values"=w358:dbl[])  [unwired: 6 in, 2 out]
          n162 = call-poly <vilib>:"NT Write Value.vi"("Numeric Array"=w358, "Name"="Drive Motors") -> ()  [unwired: 9 in, 1 out]
        }
        frame #10 {
          n163 = call <vilib>:"WPI_RobotDriveRefNum Registry Get.vi"("refnum name"="Left and Right Motors") -> ("RobotDriveDevRef"=w381:T3)  [unwired: 9 in, 1 out]
          n164 = call-poly <vilib>:"WPI_RobotDriveArcadeDrive.vi"("Y axis value"=-0.6, "X axis value"=0.0, "RobotDriveDevRef"=w381) -> ("Motor Values"=w380:dbl[], "RobotDriveDevRef"=w378:T3)  [unwired: 6 in, 1 out]
          n165 = call <vilib>:"WPI_RobotDriveDelayAndUpdateSafety.vi"("Delay (s)"=2.6, "RobotDriveDevRef"=w378) -> ("RobotDriveDevRef 2"=w373:T3)  [unwired: 8 in, 1 out]
          n166 = call-poly <vilib>:"NT Write Value.vi"("Numeric Array"=w380, "Name"="Drive Motors") -> ()  [unwired: 9 in, 1 out]
          n167 = call-poly <vilib>:"WPI_RobotDriveArcadeDrive.vi"("Y axis value"=0.0, "X axis value"=0.0, "RobotDriveDevRef"=w373) -> ("Motor Values"=w369:dbl[])  [unwired: 6 in, 2 out]
          n168 = call-poly <vilib>:"NT Write Value.vi"("Numeric Array"=w369, "Name"="Drive Motors") -> ()  [unwired: 9 in, 1 out]
        }
        frame #11 {
          n169 = call <vilib>:"WPI_RobotDriveRefNum Registry Get.vi"("refnum name"="Left and Right Motors") -> ("RobotDriveDevRef"=w394:T3)  [unwired: 9 in, 1 out]
          n170 = call-poly <vilib>:"WPI_RobotDriveArcadeDrive.vi"("Y axis value"=0.0, "X axis value"=-0.6, "RobotDriveDevRef"=w394) -> ("Motor Values"=w393:dbl[], "RobotDriveDevRef"=w391:T3)  [unwired: 6 in, 1 out]
          n171 = call <vilib>:"WPI_RobotDriveDelayAndUpdateSafety.vi"("Delay (s)"=0.37, "RobotDriveDevRef"=w391) -> ("RobotDriveDevRef 2"=w386:T3)  [unwired: 8 in, 1 out]
          n172 = call-poly <vilib>:"NT Write Value.vi"("Numeric Array"=w393, "Name"="Drive Motors") -> ()  [unwired: 9 in, 1 out]
          n173 = call-poly <vilib>:"WPI_RobotDriveArcadeDrive.vi"("Y axis value"=0.0, "X axis value"=0.0, "RobotDriveDevRef"=w386) -> ("Motor Values"=w382:dbl[])  [unwired: 6 in, 2 out]
          n174 = call-poly <vilib>:"NT Write Value.vi"("Numeric Array"=w382, "Name"="Drive Motors") -> ()  [unwired: 9 in, 1 out]
        }
        frame #12 {
          n175 = call <vilib>:"WPI_MotorControlRefNum Registry Get.vi"("refnum name"="Shooter") -> ("MotorControlDevRef"=w398:T4)  [unwired: 9 in, 1 out]
          n176 = call <vilib>:"WPI_MotorControlSetOutput.vi"("Output"=1.0, "MotorControlDevRef"=w398) -> ("MotorControlDevRef"=w395:T4)  [unwired: 7 in, 2 out]
        }
        frame #13 {
          n177 = Wait (ms)(milliseconds to wait=u32 2000) -> ()  [unwired: 1 out]
        }
        frame #14 {
          n178 = call <vilib>:"WPI_MotorControlSetOutput.vi"("Output"=0.0, "MotorControlDevRef"=w401) -> ()  [unwired: 7 in, 3 out]
        }
      }
    }
    frame "Empty" {
      # "This is some simple sample code to drive your robot curving one direction and then the other."
    }
    frame "Your Turn" {
      n179 = flat-sequence {
        tunnel: [w417] -> w412
        tunnel: w412 -> [w421]
        tunnel: [w421] -> w411
        tunnel: w411 -> [w423]
        tunnel: [w448] -> w415
        tunnel: [w447] -> w413
        tunnel: [w443] -> w404
        tunnel: [w457] -> w416
        tunnel: w415 -> [w457]
        tunnel: [w456] -> w414
        tunnel: w413 -> [w456]
        tunnel: w404 -> [w455]
        tunnel: [w455] -> w403
        tunnel: w416 -> [w462]
        tunnel: w414 -> [w461]
        tunnel: w403 -> [w459]
        tunnel: [w466] -> w408
        tunnel: [w465] -> w406
        tunnel: w408 -> [w474]
        tunnel: [w474] -> w407
        tunnel: w406 -> [w473]
        tunnel: [w473] -> w405
        tunnel: w407 -> [w477]
        tunnel: w405 -> [w476]
        tunnel: [w498] -> w409
        tunnel: [w503] -> w410
        tunnel: w409 -> [w503]
        tunnel: w410 -> [w504]
        frame #0 {
          n180 = call <vilib>:"WPI_MotorControlRefNum Registry Get.vi"("refnum name"="Shooter") -> ("MotorControlDevRef"=w420:T4)  [unwired: 9 in, 1 out]
          n181 = call <vilib>:"WPI_MotorControlSetOutput.vi"("Output"=1.0, "MotorControlDevRef"=w420) -> ("MotorControlDevRef"=w417:T4)  [unwired: 7 in, 2 out]
        }
        frame #1 {
          n182 = Wait (ms)(milliseconds to wait=u32 2000) -> ()  [unwired: 1 out]
        }
        frame #2 {
          n183 = call <vilib>:"WPI_MotorControlSetOutput.vi"("Output"=0.0, "MotorControlDevRef"=w423) -> ()  [unwired: 7 in, 3 out]
        }
        frame #3 {
          w425 = "RobotDrive Motors" ("Name")
          # "stand still"
          # "other way for 0.5 second"
          # "turn for 1 second"
          n184 = call <vilib>:"WPI_RobotDriveRefNum Registry Get.vi"("refnum name"="Left and Right Motors") -> ("RobotDriveDevRef"=w435:T3)  [unwired: 1 in, 9 out]
          n185 = call-poly <vilib>:"WPI_RobotDriveArcadeDrive.vi"("Y axis value"=-0.7 ("X axis value"), "X axis value"=0.5, "RobotDriveDevRef"=w435) -> ("Motor Values"=w441:dbl[], "RobotDriveDevRef"=w438:T3)  [unwired: 1 in, 6 out]
          n186 = call-poly <vilib>:"NT Write Value.vi"("Numeric Array"=w441, "Name"=w425) -> ()  [unwired: 9 in, 1 out]
          n187 = call <vilib>:"WPI_RobotDriveDelayAndUpdateSafety.vi"("Delay (s)"=2.0, "RobotDriveDevRef"=w438) -> ("RobotDriveDevRef 2"=w442:T3)  [unwired: 8 in, 1 out]
          n188 = call-poly <vilib>:"WPI_RobotDriveArcadeDrive.vi"("Y axis value"=-0.5 ("X axis value"), "X axis value"=0.7, "RobotDriveDevRef"=w442) -> ("Motor Values"=w440:dbl[], "RobotDriveDevRef"=w437:T3)  [unwired: 1 in, 6 out]
          n189 = call-poly <vilib>:"NT Write Value.vi"("Numeric Array"=w440, "Name"=w425) -> ()  [unwired: 9 in, 1 out]
          n190 = call <vilib>:"WPI_RobotDriveDelayAndUpdateSafety.vi"("Delay (s)"=2.0, "RobotDriveDevRef"=w437) -> ("RobotDriveDevRef 2"=w436:T3)  [unwired: 8 in, 1 out]
          n191 = call-poly <vilib>:"WPI_RobotDriveArcadeDrive.vi"("Y axis value"=0.0 ("X axis value"), "X axis value"=0.0, "RobotDriveDevRef"=w436) -> ("Motor Values"=w439:dbl[])  [unwired: 1 in, 7 out]
          n192 = call-poly <vilib>:"NT Write Value.vi"("Numeric Array"=w439, "Name"=w425) -> ()  [unwired: 9 in, 1 out]
        }
        frame #4 {
          n193 = call <vilib>:"WPI_MotorControlRefNum Registry Get.vi"("refnum name"="Window 2") -> ("MotorControlDevRef"=w451:T4)  [unwired: 9 in, 1 out]
          n194 = call <vilib>:"WPI_MotorControlRefNum Registry Get.vi"("refnum name"="Window 1") -> ("MotorControlDevRef"=w453:T4)  [unwired: 9 in, 1 out]
          n195 = call <vilib>:"WPI_MotorControlRefNum Registry Get.vi"("refnum name"="Intake Wheel") -> ("MotorControlDevRef"=w445:T4)  [unwired: 9 in, 1 out]
          n196 = call <vilib>:"WPI_MotorControlSetOutput.vi"("Output"=0.5, "MotorControlDevRef"=w451) -> ("MotorControlDevRef"=w447:T4)  [unwired: 7 in, 2 out]
          n197 = call <vilib>:"WPI_MotorControlSetOutput.vi"("Output"=0.5, "MotorControlDevRef"=w453) -> ("MotorControlDevRef"=w448:T4)  [unwired: 7 in, 2 out]
          n198 = call <vilib>:"WPI_MotorControlSetOutput.vi"("Output"=1.0, "MotorControlDevRef"=w445) -> ("MotorControlDevRef"=w443:T4)  [unwired: 7 in, 2 out]
        }
        frame #5 {
          n199 = Wait (ms)(milliseconds to wait=u32 3000) -> ()  [unwired: 1 out]
        }
        frame #6 {
          n200 = call <vilib>:"WPI_MotorControlSetOutput.vi"("Output"=0.0, "MotorControlDevRef"=w459) -> ()  [unwired: 7 in, 3 out]
          n201 = call <vilib>:"WPI_MotorControlSetOutput.vi"("Output"=0.0, "MotorControlDevRef"=w462) -> ()  [unwired: 7 in, 3 out]
          n202 = call <vilib>:"WPI_MotorControlSetOutput.vi"("Output"=0.0, "MotorControlDevRef"=w461) -> ()  [unwired: 7 in, 3 out]
        }
        frame #7 {
          n203 = call <vilib>:"WPI_MotorControlRefNum Registry Get.vi"("refnum name"="Window 2") -> ("MotorControlDevRef"=w469:T4)  [unwired: 9 in, 1 out]
          n204 = call <vilib>:"WPI_MotorControlRefNum Registry Get.vi"("refnum name"="Window 1") -> ("MotorControlDevRef"=w471:T4)  [unwired: 9 in, 1 out]
          n205 = call <vilib>:"WPI_MotorControlSetOutput.vi"("Output"=-0.5, "MotorControlDevRef"=w469) -> ("MotorControlDevRef"=w465:T4)  [unwired: 7 in, 2 out]
          n206 = call <vilib>:"WPI_MotorControlSetOutput.vi"("Output"=-0.5, "MotorControlDevRef"=w471) -> ("MotorControlDevRef"=w466:T4)  [unwired: 7 in, 2 out]
        }
        frame #8 {
          n207 = Wait (ms)(milliseconds to wait=u32 3000) -> ()  [unwired: 1 out]
        }
        frame #9 {
          n208 = call <vilib>:"WPI_MotorControlSetOutput.vi"("Output"=0.0, "MotorControlDevRef"=w477) -> ()  [unwired: 7 in, 3 out]
          n209 = call <vilib>:"WPI_MotorControlSetOutput.vi"("Output"=0.0, "MotorControlDevRef"=w476) -> ()  [unwired: 7 in, 3 out]
        }
        frame #10 {
          w480 = "RobotDrive Motors" ("Name")
          # "stand still"
          # "other way for 0.5 second"
          # "turn for 1 second"
          n210 = call <vilib>:"WPI_RobotDriveRefNum Registry Get.vi"("refnum name"="Left and Right Motors") -> ("RobotDriveDevRef"=w497:T3)  [unwired: 1 in, 9 out]
          n211 = call-poly <vilib>:"WPI_RobotDriveArcadeDrive.vi"("Y axis value"=-0.7 ("X axis value"), "X axis value"=0.5, "RobotDriveDevRef"=w497) -> ("Motor Values"=w491:dbl[], "RobotDriveDevRef"=w494:T3)  [unwired: 1 in, 6 out]
          n212 = call-poly <vilib>:"NT Write Value.vi"("Numeric Array"=w491, "Name"=w480) -> ()  [unwired: 9 in, 1 out]
          n213 = call <vilib>:"WPI_RobotDriveDelayAndUpdateSafety.vi"("Delay (s)"=2.0, "RobotDriveDevRef"=w494) -> ("RobotDriveDevRef 2"=w490:T3)  [unwired: 8 in, 1 out]
          n214 = call-poly <vilib>:"WPI_RobotDriveArcadeDrive.vi"("Y axis value"=-0.5 ("X axis value"), "X axis value"=0.7, "RobotDriveDevRef"=w490) -> ("Motor Values"=w492:dbl[], "RobotDriveDevRef"=w495:T3)  [unwired: 1 in, 6 out]
          n215 = call-poly <vilib>:"NT Write Value.vi"("Numeric Array"=w492, "Name"=w480) -> ()  [unwired: 9 in, 1 out]
          n216 = call <vilib>:"WPI_RobotDriveDelayAndUpdateSafety.vi"("Delay (s)"=2.0, "RobotDriveDevRef"=w495) -> ("RobotDriveDevRef 2"=w496:T3)  [unwired: 8 in, 1 out]
          n217 = call-poly <vilib>:"WPI_RobotDriveArcadeDrive.vi"("Y axis value"=0.0 ("X axis value"), "X axis value"=0.0, "RobotDriveDevRef"=w496) -> ("Motor Values"=w493:dbl[])  [unwired: 1 in, 7 out]
          n218 = call-poly <vilib>:"NT Write Value.vi"("Numeric Array"=w493, "Name"=w480) -> ()  [unwired: 9 in, 1 out]
        }
        frame #11 {
          n219 = call <vilib>:"WPI_MotorControlRefNum Registry Get.vi"("refnum name"="Shooter") -> ("MotorControlDevRef"=w501:T4)  [unwired: 9 in, 1 out]
          n220 = call <vilib>:"WPI_MotorControlSetOutput.vi"("Output"=1.0, "MotorControlDevRef"=w501) -> ("MotorControlDevRef"=w498:T4)  [unwired: 7 in, 2 out]
        }
        frame #12 {
          n221 = Wait (ms)(milliseconds to wait=u32 2000) -> ()  [unwired: 1 out]
        }
        frame #13 {
          n222 = call <vilib>:"WPI_MotorControlSetOutput.vi"("Output"=0.0, "MotorControlDevRef"=w504) -> ()  [unwired: 7 in, 3 out]
        }
      }
    }
  }
